vi "Set Pif DO.vi"(9 "Value":bool, 10 "PifChn":u16, 11 "index":u16) -> (3 "function return":bool)   [LabVIEW 2025, in "ExtremelyEpicImagerIPC2.lvlib"]
doc: "IMAGERIPC_API bool WINAPI SetPifDO(WORD index, WORD PifChn, bool Value);"
uses:
  ExtremelyEpicImagerIPC2.lvlib
  ImagerIPC2.dll
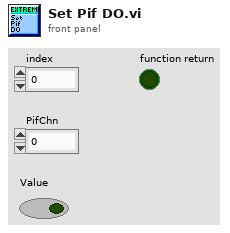
[diagram p1: front panel]
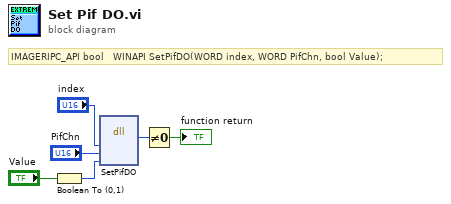
[diagram p0: block diagram]
diagram:
  # "IMAGERIPC_API bool \t WINAPI SetPifDO(WORD index, WORD PifChn, bool Value);"
  n1 = Boolean To (0,1)(Boolean="Value") -> (0, 1=w1:i16)
  n2 = dll-call lib="C:/Users/mayhe/OneDrive/Documents/GitHub/In-situ-monitoring-of-powder-bed-fusion-additive-manufacturing/system_development/Orichalcum/v0.2/Software_design/thermal-camera/VI/Connect SDK/ImagerIPC2.*" fn="SetPifDO"("index"="index", "PifChn"="PifChn", "Value"=w1) -> (w5:u8)  [unwired: 6 in, 2 out]
  n3 = Not Equal To 0?(x=w5) -> (x != 0?=→"function return":bool)
